vi "Fetch Room Sizes.vi"(0 "Rooms Manager Model in":refnum<class "Rooms Manager Model.lvclass">, 11 "error in (no error)":errorcluster) -> (4 "Rooms Manager Model out":refnum<class "Rooms Manager Model.lvclass">, 15 "error out":errorcluster)   [LabVIEW 2023, in "Rooms Manager Model.lvlib" / "Rooms Manager Model.lvclass"]
uses:
  Rooms Manager Model.lvclass
  <vilib>/ActorFramework/Actor/Actor.lvclass/Actor.ctl
  <vilib>/ActorFramework/Message Enqueuer/Message Enqueuer.lvclass/Message Enqueuer.ctl
  Rooms Manager Model.lvclass/Rooms Manager Model.ctl
  Guest Manager Model/Guest Manager Model Messages/Update room Size Msg/Update room Size Msg.lvclass/Update room Size Msg.ctl
  <vilib>/ActorFramework/Message Enqueuer/Init from Existing Queue.vi
  <vilib>/ActorFramework/Message Enqueuer/Enqueue.vi
  Guest Manager Model/Guest Manager Model Messages/Update room Size Msg/Update room Size Msg.lvclass
  C:/Program Files/National Instruments/LabVIEW 2023/vi.lib/ActorFramework/Message/Message.lvclass
  <vilib>/ActorFramework/Message Priority Queue/Priority Enqueue.vi
  <vilib>/ActorFramework/Message Enqueuer/Message Enqueuer.lvclass
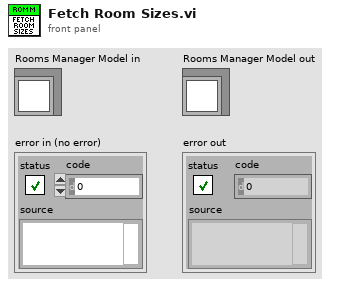
[diagram p1: front panel]
types:
  T1 = typedef "Central Data Manager.lvlib/Central Data Manager.lvclass/Room Size Details.ctl" = cluster{"Size":string, "Cost Per Day (Rs)":u32, "Occupancy Limit (Adult)":u32, "Occupancy Limit (Children)":u32}
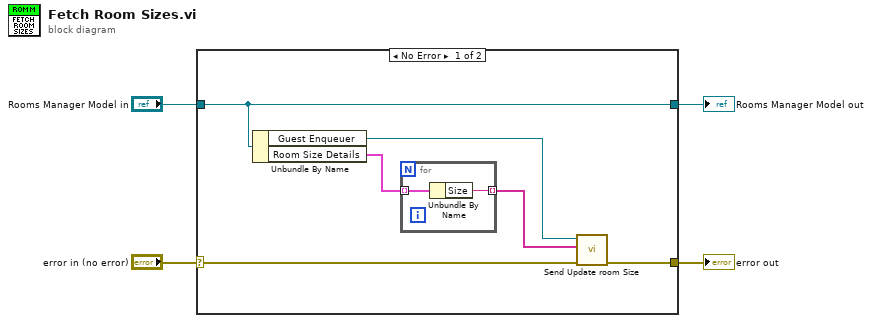
[diagram p0: block diagram]
diagram:
  n1 = case shown="No Error" "error in (no error)" {
    selector: "error in (no error)" -> [w10 w13]
    tunnel: [w9 w13] -> w4
    tunnel: "Rooms Manager Model in" -> [w5 w14]
    tunnel: [w5 w14] -> w1
    frame No Error {
      n2 = Unbundle By Name(w5) -> ("Guest Enqueuer"=w6:refnum<class "Message Enqueuer.lvclass">, "Room Size Details"=w8:T1[])
      n3 = for {
        tunnel: w8 -> [w12] mode=indexing
        tunnel: [w11] -> w7 mode=indexing
        n4 = Unbundle By Name(w12) -> ("Size"=w11:string)
      }
      n5 = call "Send Update room Size.vi"("error in (no error)"=w10, "Room Sizes"=w7, "Message Enqueuer"=w6) -> ("error out"=w9:errorcluster)  [unwired: 7 in, 1 out]
    }
    frame Error {
    }
  }
  "error out" <- w4
  "Rooms Manager Model out" <- w1
